vi "FIFO Last Measurement Wfm Results.vi"(8 "Channels Per Record":i32=1, 9 "Record Upper Limit":i32=10, 10 "New Data":T1, 11 "measurement results in":T2 {"Actual Record Length" format="%#_6p Samples"; "Actual Record Duration" format="%#_6ps"; "Actual Sample Rate" format="%#_6pHz"}) -> (3 "measurement results out":T2 {"Actual Record Length" format="%#_6p Samples"; "Actual Record Duration" format="%#_6ps"; "Actual Sample Rate" format="%#_6pHz"})   [LabVIEW 2025, in "Ni-Scope-Multirecords.lvclass"]
uses:
  Ni-Scope-Multirecords.lvclass
  Ni-Scope-Multirecords.lvclass/Ni-Scope-Multirecords.ctl
  Measurement Results.ctl
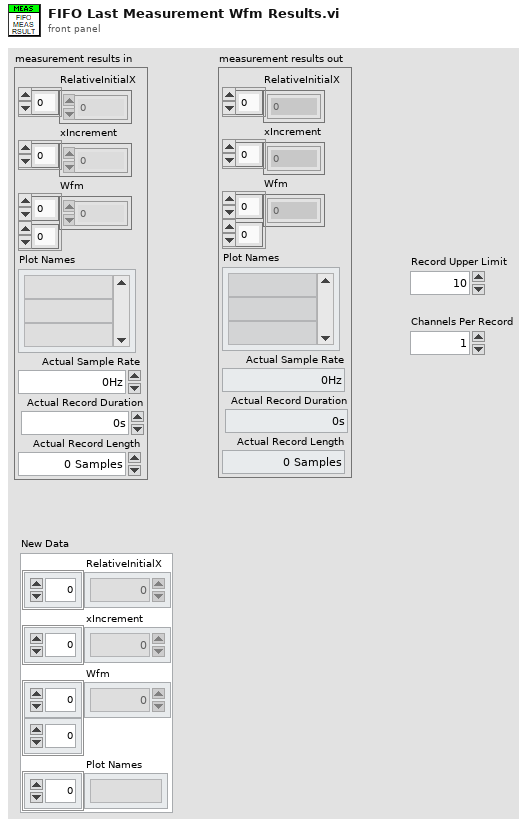
[diagram p1: front panel]
types:
  T1 = cluster{"RelativeInitialX":dbl[], "xIncrement":dbl[], "Wfm":dbl[][], "Plot Names":string[]}
  T2 = typedef "Ni-Scope-Multirecords.lvclass/Measurement Results.ctl" = cluster{"RelativeInitialX":dbl[], "xIncrement":dbl[], "Wfm":dbl[][], "Plot Names":string[], "Actual Sample Rate":dbl, "Actual Record Duration":dbl, "Actual Record Length":dbl}
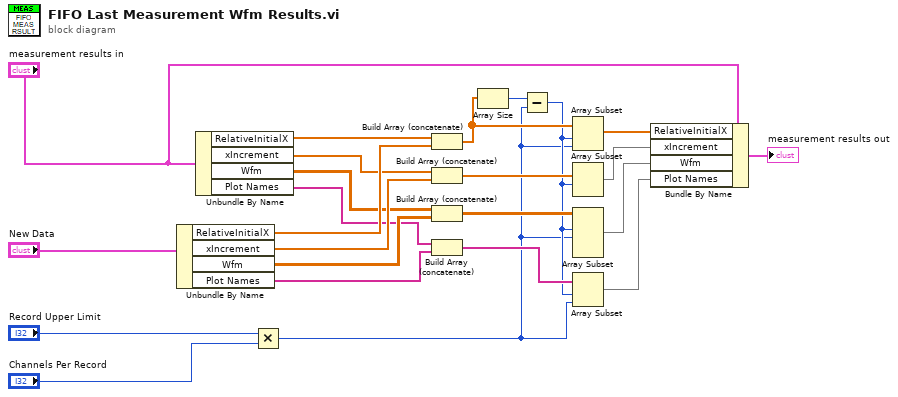
[diagram p0: block diagram]
diagram:
  n1 = Unbundle By Name("New Data") -> ("RelativeInitialX"=w22:dbl[], "xIncrement"=w20:dbl[], "Wfm"=w18:dbl[][], "Plot Names"=w16:string[])
  n2 = Unbundle By Name("measurement results in") -> ("RelativeInitialX"=w24:dbl[], "xIncrement"=w21:dbl[], "Wfm"=w19:dbl[][], "Plot Names"=w17:string[])
  n3 = Multiply(x="Record Upper Limit", y="Channels Per Record") -> (x*y=w2:i32)
  n4 = Build Array (concatenate)(w24, w22) -> (w15:dbl[])
  n5 = Build Array (concatenate)(w21, w20) -> (w13:dbl[])
  n6 = Build Array (concatenate)(w19, w18) -> (w12:dbl[][])
  n7 = Build Array (concatenate)(w17, w16) -> (w11:string[])
  n8 = Array Size(array=w15) -> (size(s)=w14:i32)
  n9 = Subtract(x=w14, y=w2) -> (x-y=w10:i32)
  n10 = Array Subset(array=w15, index=w10, length=w2) -> (w7:dbl[])
  n11 = Array Subset(array=w13, index=w10) -> (w6:dbl[])  [unwired: 1 in]
  n12 = Array Subset(array=w12, index (row)=w10, length (row)=w2) -> (w5:dbl[][])  [unwired: 2 in]
  n13 = Array Subset(array=w11, index=w10, length=w2) -> (w4:string[])
  n14 = Bundle By Name(cluster="measurement results in", "RelativeInitialX"=w7, "xIncrement"=w6, "Wfm"=w5, "Plot Names"=w4) -> (→"measurement results out":T2)
